vi "LKS340 set P.vi"(1 "error in":errorcluster, 2 "Set point":dbl format="%.2f", 3 "GPIB Adress":i16) -> (0 "error out":errorcluster)   [LabVIEW 2014]
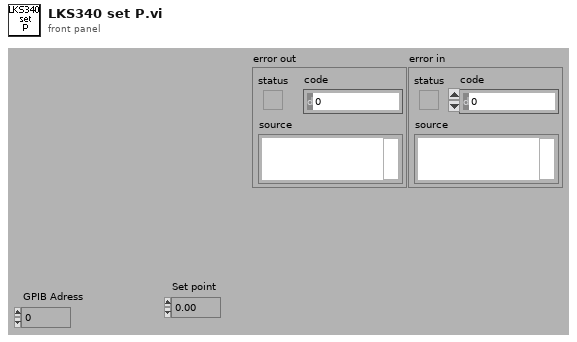
[diagram p1: front panel]
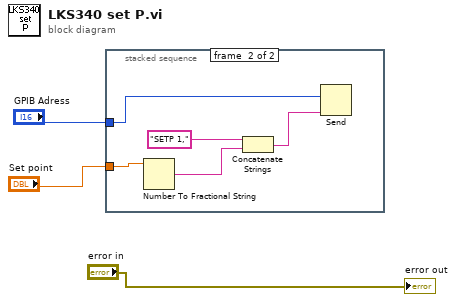
[diagram p0: block diagram]
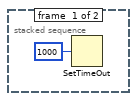
[diagram p2: hidden frame]
diagram:
  n1 = stacked-sequence {
    tunnel: "GPIB Adress" -> [_ w9]
    tunnel: "Set point" -> [_ w6]
    frame #0 {
      n2 = SetTimeOut(1:1000 ("new timeout (10000)")) -> ()  [unwired: 1 out]
    }
    frame #1 {
      n3 = Number To Fractional String(number=w6) -> (F-format string=w8:string)  [unwired: 3 in]
      n4 = Concatenate Strings("SETP 1," ("data string"), w8) -> (w5:string)
      n5 = Send(2:w9, 5:w5) -> ()  [unwired: 3 in, 3 out]
    }
  }
  "error out" <- "error in"
